vi "Wait(Second).vi"(8 "Error In":errorcluster, 11 "等待秒數(3000毫秒)":dbl=750.0) -> (0 "Error Out":errorcluster)   [LabVIEW 2019]
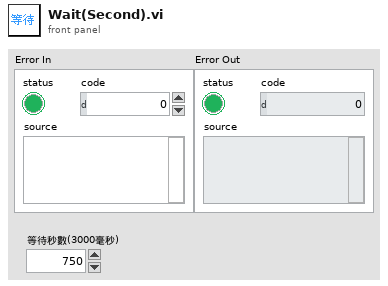
[diagram p1: front panel]
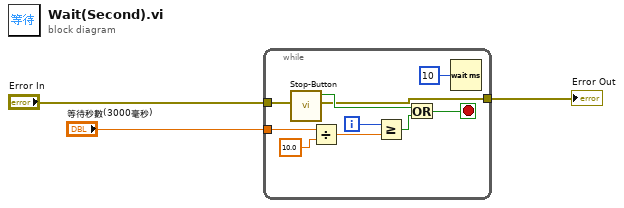
[diagram p0: block diagram]
diagram:
  n1 = while {
    tunnel: "等待秒數(3000毫秒)" -> [w11]
    tunnel: "Error In" -> [w4]
    tunnel: [w5] -> w3
    i -> [w8]
    stop <- w12 stop-if-true
    n2 = call "Stop-Button.vi"("Error In"=w4) -> ("Error Out"=w5:errorcluster, "顯示按下?"=w6:bool)  [unwired: 9 in]
    n3 = Divide(x=w11, y=10.0) -> (x/y=w7:dbl)
    n4 = Greater Or Equal?(x=w8, y=w7) -> (x >= y?=w9:bool)
    n5 = Or(x=w6, y=w9) -> (x .or. y?=w12:bool)
    n6 = Wait (ms)(milliseconds to wait=u32 10) -> ()  [unwired: 1 out]
  }
  "Error Out" <- w3
